vi "sub build keyword value.vi"(6 "EOF":string, 7 "SOF":string, 8 "error in":errorcluster, 10 "value":string[](array[string]), 11 "keyword":string[](array[string])) -> (0 "error out":errorcluster, 3 "keyword value string":string)   [LabVIEW 2018, in "Frame Analizer.lvclass"]
uses:
  Frame Analizer.lvclass
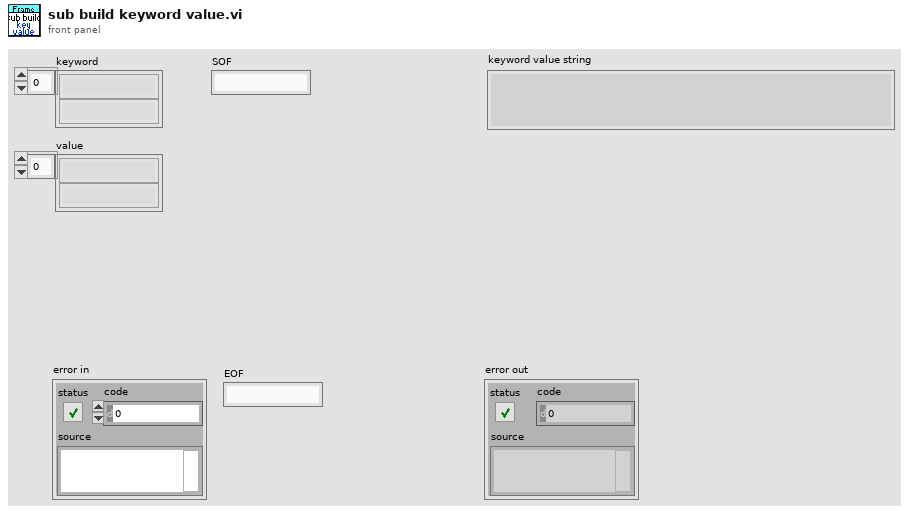
[diagram p1: front panel]
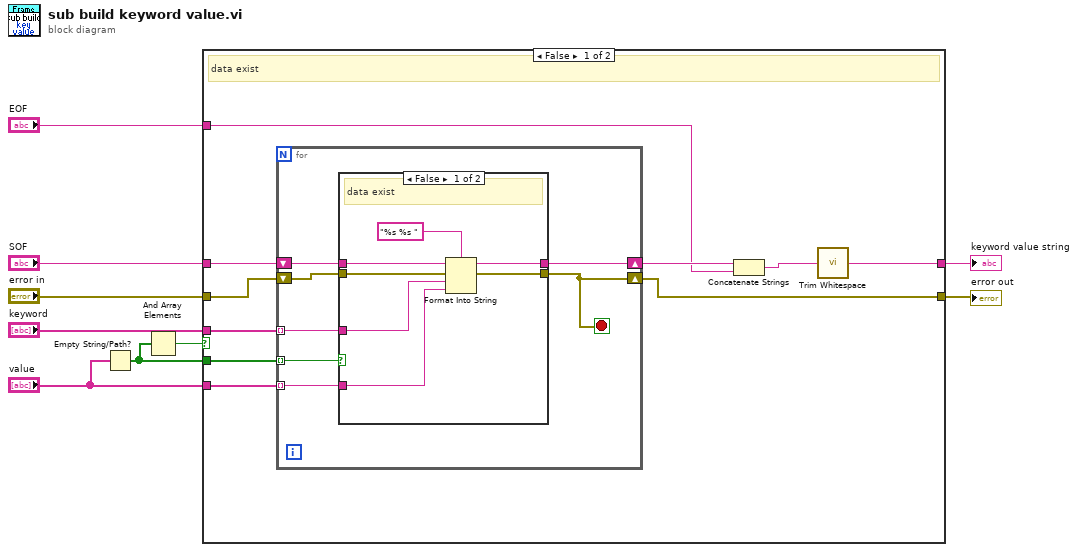
[diagram p0: block diagram]
diagram:
  n1 = Empty String/Path?(string/path="value") -> (empty?=w6:bool[])
  n2 = And Array Elements(Boolean array=w6) -> (logical AND=w5:bool)
  n3 = case shown="False" w5 {
    tunnel: "error in" -> [w19 w36]
    tunnel: [w18 w36] -> w8
    tunnel: "keyword" -> [w17 _]
    tunnel: "value" -> [w16 _]
    tunnel: w6 -> [w15 _]
    tunnel: [w10 _] -> w4
    tunnel: "SOF" -> [w12 _]
    tunnel: "EOF" -> [w11 _]
    frame False {
      # "data exist"
      n4 = for {
        tunnel: w17 -> [w25] mode=indexing
        shift-right: [w24] -> w14
        shift-left: w12 -> [w26]
        shift-right: [w22] -> w18
        shift-left: w19 -> [w23]
        tunnel: w16 -> [w21] mode=indexing
        tunnel: w15 -> [w20] mode=indexing
        stop <- w22 stop-if-true
        n5 = case shown="False" w20 {
          tunnel: w26 -> [w33 w35]
          tunnel: w25 -> [w32 _]
          tunnel: [w30 w35] -> w24
          tunnel: w23 -> [w29 w34]
          tunnel: [w28 w34] -> w22
          tunnel: w21 -> [w27 _]
          frame False {
            # "data exist"
            n6 = Format Into String(format string="%s %s ", initial string=w33, error in=w29, w32, w27) -> (resulting string=w30:string, error out=w28:errorcluster)
          }
          frame True {
            # "no data, skip"
          }
        }
      }
      n7 = Concatenate Strings(w14, w11) -> (w13:string)
      n8 = call <vilib>:"Trim Whitespace.vi"("string"=w13) -> ("trimmed string"=w10:string)  [unwired: 1 in]
    }
    frame True {
      # "no data, skip"
    }
  }
  "keyword value string" <- w4
  "error out" <- w8
